vi "Get Channel Data.vi"(5 "Static File Structure":bool, 6 "Tree Location":string, 7 "Relative File Paths":string[](array[string]), 8 "error in (no error)":errorcluster, 9 "Hierarchy":string[](array[string]), 10 "Data Directory":path, 11 "TreeControl in":refnum<vi>) -> (0 "error out":errorcluster, 3 "Tree Selection Data Array":T1[](array[typedef]))   [LabVIEW 2017, in "XTree.xctl"]
doc: "Gets information of all of the channels under a location in the tree."
uses:
  <vilib>/addons/_NIFileIO/XTree/XTree.xctl
  <vilib>/addons/_NIFileIO/XTree/Controls/Tree Selection Data.ctl
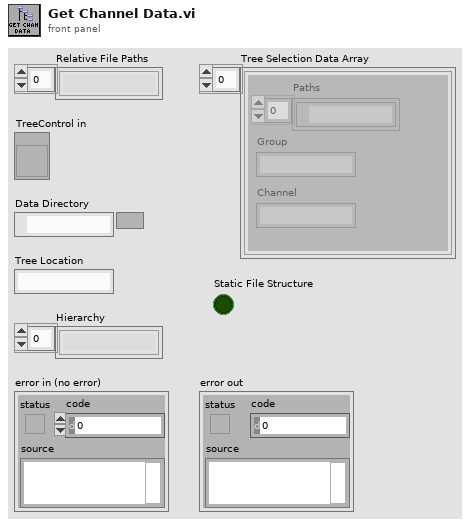
[diagram p1: front panel]
types:
  T1 = typedef "XTree.xctl/Tree Selection Data.ctl" = cluster{"Paths":path[], "Group":string, "Channel":string}
  T2 = enum16{"open", "open or create", "create or replace", "create", "open (read-only)"}
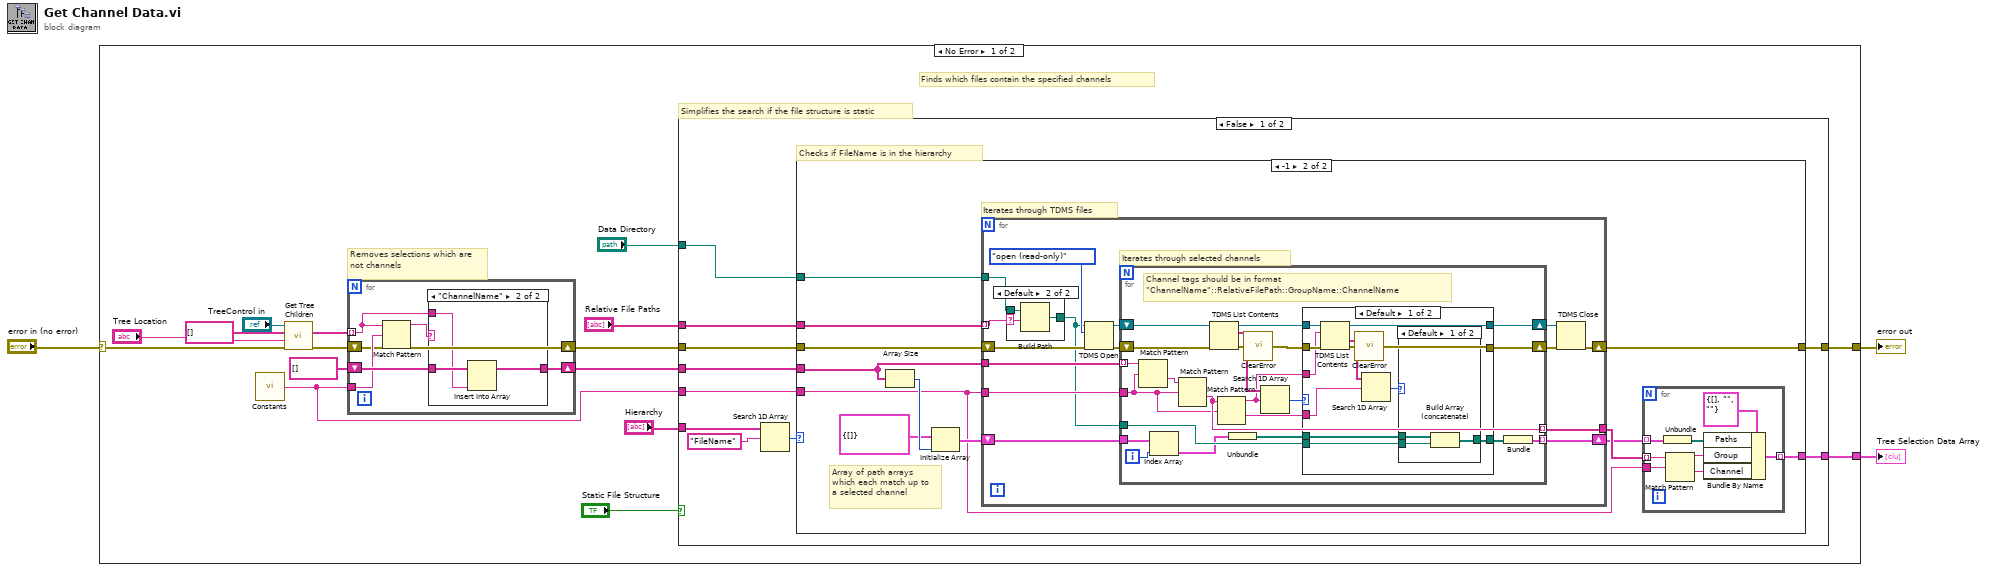
[diagram p0: block diagram]
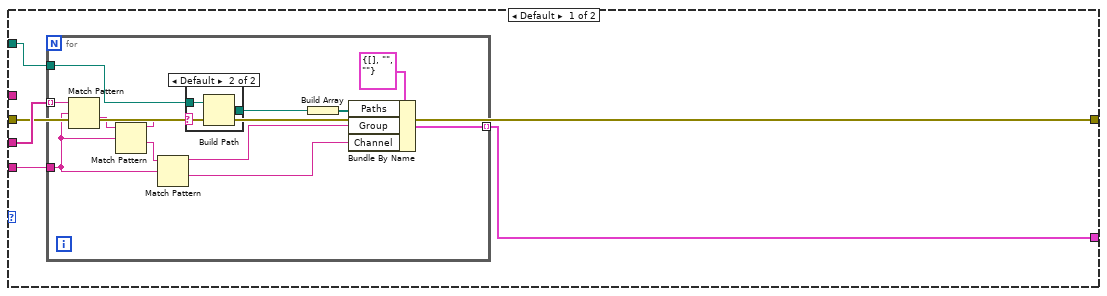
[diagram p2: hidden frame]
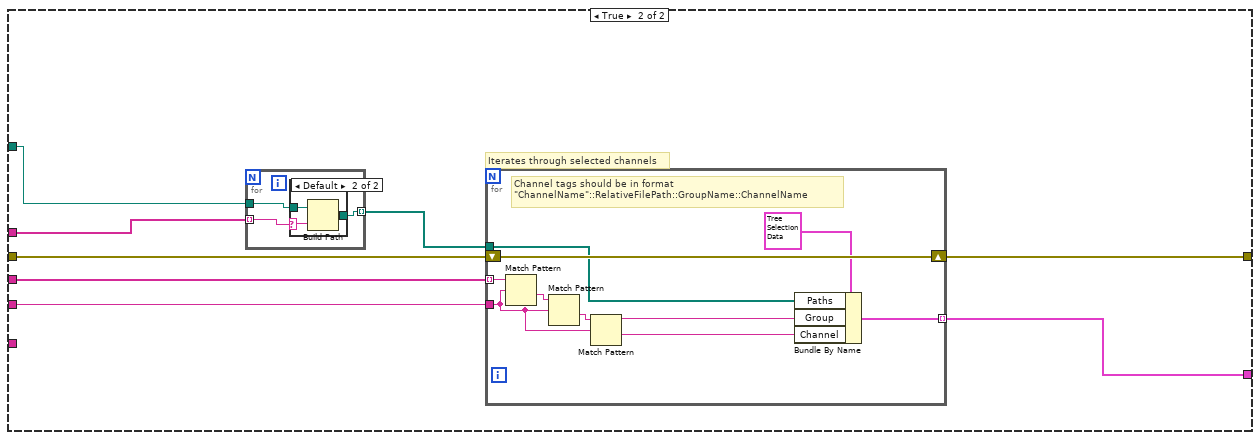
[diagram p7: hidden frame]
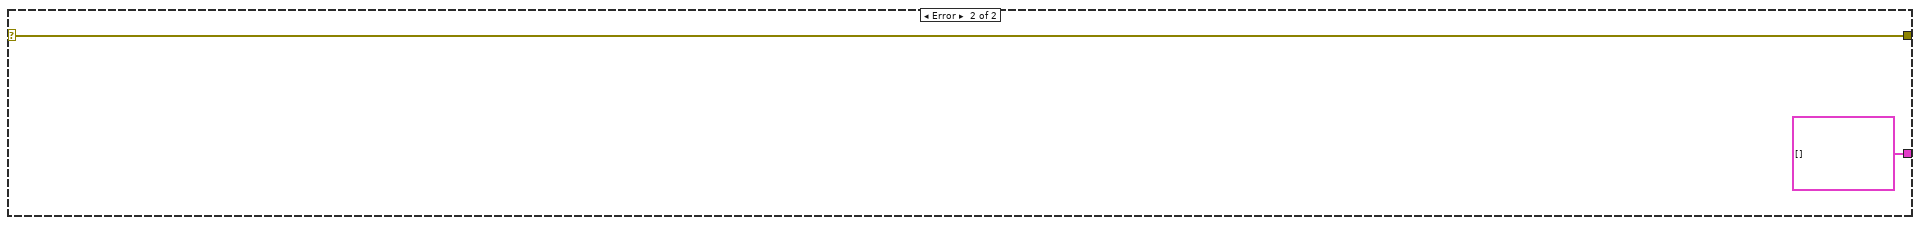
[diagram p10: hidden frame]
diagram:
  n1 = case shown="No Error" "error in (no error)" {
    selector: "error in (no error)" -> [w5 w167]
    tunnel: [w18 w167] -> w3
    tunnel: [w4 T1[] []] -> w1
    frame No Error {
      # "Simplifies the search if the file structure is static"
      # "Finds which files contain the specified channels"
      # "Removes selections which are not channels"
      n2 = call <vilib>:"Constants.vi"() -> ("String Delimeter"=w10:string)  [unwired: 5 in]
      n3 = call <vilib>:"Get Tree Children.vi"("error in (no error)"=w5, "Parent Tag"="Tree Location", "Child Tags In"=string[] [], "File Contents Tree"="TreeControl in") -> ("error out"=w11:errorcluster, "Child Tags Out"=w13:string[])  [unwired: 6 in]
      n4 = for {
        tunnel: w13 -> [w159] mode=indexing
        shift-right: [w160] -> w9
        shift-left: string[] [] -> [w161]
        shift-right: [w156] -> w8
        shift-left: w11 -> [w156]
        tunnel: w10 -> [w158]
        n5 = Match Pattern(string=w159, regular expression=w158) -> (before substring=w157:string)  [unwired: 1 in, 3 out]
        n6 = case shown="\"ChannelName\"" w157 {
          tunnel: w161 -> [w162 w165]
          tunnel: [w162 w164] -> w160
          tunnel: w159 -> [_ w163]
          frame Default {
          }
          frame "ChannelName" {
            n7 = Insert Into Array(array=w165, new element=w163) -> (w164:string[])  [unwired: 1 in]
          }
        }
      }
      n8 = case shown="False" "Static File Structure" {
        tunnel: "Hierarchy" -> [w27 _]
        tunnel: [w26 w132] -> w4
        tunnel: [w25 w138] -> w18
        tunnel: "Data Directory" -> [w24 w137]
        tunnel: "Relative File Paths" -> [w23 w136]
        tunnel: w10 -> [w22 w135]
        tunnel: w9 -> [w21 w134]
        tunnel: w8 -> [w20 w131]
        frame False {
          # "Checks if FileName is in the hierarchy"
          n9 = Search 1D Array(1D array=w27, element="FileName") -> (index of element=w29:i32)  [unwired: 1 in]
          n10 = case shown="-1" w29 {
            tunnel: w23 -> [_ w62]
            tunnel: w20 -> [w30 w61]
            tunnel: w21 -> [w34 w57]
            tunnel: w24 -> [w32 w54]
            tunnel: [w30 w53] -> w25
            tunnel: [w31 w52] -> w26
            tunnel: w22 -> [w33 w51]
            frame Default {
              n11 = for {
                tunnel: w34 -> [w46] mode=indexing
                tunnel: w33 -> [w41]
                tunnel: w32 -> [w37]
                tunnel: [w43] -> w31 mode=indexing
                n12 = Match Pattern(string=w46, regular expression=w41) -> (after substring=w45:string)  [unwired: 1 in, 3 out]
                n13 = Match Pattern(string=w45, regular expression=w41) -> (before substring=w36:string, after substring=w42:string)  [unwired: 1 in, 2 out]
                n14 = Match Pattern(string=w42, regular expression=w41) -> (before substring=w40:string, after substring=w39:string)  [unwired: 1 in, 2 out]
                n15 = case shown="Default" w36 {
                  selector: w36 -> [_ w48]
                  tunnel: w37 -> [w47 w50]
                  tunnel: [w47 w49] -> w35
                  frame "" {
                  }
                  frame Default {
                    n16 = Build Path(base path=w50, name or relative path=w48) -> (appended path=w49:path)
                  }
                }
                n17 = Build Array(w35) -> (w44:path[])
                n18 = Bundle By Name(cluster=T1 {"Paths"=[], "Group"="", "Channel"=""} ("Tree Selection Data"), "Paths"=w44, "Group"=w40, "Channel"=w39) -> (w43:T1)
              }
            }
            frame -1 {
              # "Array of path arrays which each match up to a selected channel"
              # "Iterates through TDMS files"
              n19 = Array Size(array=w57) -> (size(s)=w58:i32)
              n20 = Initialize Array(cluster{path[]} {[]}, w58) -> (w55:cluster{path[]}[])
              n21 = for {
                tunnel: w62 -> [w71] mode=indexing
                shift-right: [w84] -> w53
                shift-left: w61 -> [w74]
                tunnel: w57 -> [w82]
                tunnel: w51 -> [w79]
                shift-right: [w77] -> w59
                shift-left: w55 -> [w78]
                tunnel: [w76] -> w60
                tunnel: w54 -> [w73]
                # "Iterates through selected channels"
                n22 = case shown="Default" w71 {
                  selector: w71 -> [_ w87]
                  tunnel: w73 -> [w86 w89]
                  tunnel: [w86 w88] -> w72
                  frame "" {
                  }
                  frame Default {
                    n23 = Build Path(base path=w89, name or relative path=w87) -> (appended path=w88:path)
                  }
                }
                n24 = TDMS Open(8:w74, 10:T2."open (read-only)" ("operation (0:open)"), 11:w72) -> (0:w75:errorcluster, 3:w80:refnum<k34>)  [unwired: 4 in]
                n25 = for {
                  tunnel: w72 -> [w111]
                  shift-right: [w109] -> w85
                  shift-left: w75 -> [w98]
                  tunnel: w82 -> [w110] mode=indexing
                  tunnel: w79 -> [w100]
                  tunnel: w78 -> [w105]
                  tunnel: [w106] -> w77 mode=indexing
                  tunnel: [w101] -> w76 mode=indexing
                  shift-right: [w91] -> w83
                  shift-left: w80 -> [w99]
                  i -> [w104]
                  # "Channel tags should be in format \n\"ChannelName\"::RelativeFilePath::GroupName::ChannelName"
                  n26 = Match Pattern(string=w110, regular expression=w100) -> (after substring=w102:string)  [unwired: 1 in, 3 out]
                  n27 = Index Array(array=w105, index=w104) -> (element=w103:cluster{path[]})
                  n28 = Match Pattern(string=w102, regular expression=w100) -> (after substring=w101:string)  [unwired: 1 in, 3 out]
                  n29 = TDMS List Contents(4:w98, 7:w99) -> (0:w90:errorcluster, 2:w96:string[], 3:w93:refnum<k34>)  [unwired: 1 in, 1 out]
                  n30 = Match Pattern(string=w101, regular expression=w100) -> (before substring=w94:string, after substring=w95:string)  [unwired: 1 in, 2 out]
                  n31 = Unbundle(w103) -> (w108:path[])
                  n32 = call <vilib>:"ClearError.vi"("error in (no error)"=w90) -> ("error out"=w92:errorcluster)
                  n33 = Search 1D Array(1D array=w96, element=w94) -> (index of element=w97:i32)  [unwired: 1 in]
                  n34 = case shown="Default" w97 {
                    tunnel: [w114 w129] -> w109
                    tunnel: w108 -> [w117 w130]
                    tunnel: w111 -> [w115 _]
                    tunnel: [w116 w130] -> w107
                    tunnel: w95 -> [w118 _]
                    tunnel: w94 -> [w120 _]
                    tunnel: w93 -> [w123 w128]
                    tunnel: w92 -> [w122 w129]
                    tunnel: [w113 w128] -> w91
                    frame Default {
                      n35 = TDMS List Contents(4:w122, 6:w120, 7:w123) -> (0:w112:errorcluster, 1:w119:string[], 3:w113:refnum<k34>)  [unwired: 1 out]
                      n36 = call <vilib>:"ClearError.vi"("error in (no error)"=w112) -> ("error out"=w114:errorcluster)
                      n37 = Search 1D Array(1D array=w119, element=w118) -> (index of element=w121:i32)  [unwired: 1 in]
                      n38 = case shown="Default" w121 {
                        tunnel: w117 -> [w126 w127]
                        tunnel: [w125 w127] -> w116
                        tunnel: w115 -> [w124 _]
                        frame Default {
                          n39 = Build Array (concatenate)(w126, w124) -> (w125:path[])
                        }
                        frame -1 {
                        }
                      }
                    }
                    frame -1 {
                    }
                  }
                  n40 = Bundle(w107) -> (w106:cluster{path[]})  [unwired: 1 in]
                }
                n41 = TDMS Close(8:w85, 11:w83) -> (0:w84:errorcluster)  [unwired: 1 out]
              }
              n42 = for {
                tunnel: w60 -> [w70] mode=indexing
                tunnel: w51 -> [w69]
                tunnel: w59 -> [w68] mode=indexing
                tunnel: [w66] -> w52 mode=indexing
                n43 = Unbundle(w68) -> (w67:path[])
                n44 = Match Pattern(string=w70, regular expression=w69) -> (before substring=w65:string, after substring=w64:string)  [unwired: 1 in, 2 out]
                n45 = Bundle By Name(cluster=T1 {"Paths"=[], "Group"="", "Channel"=""} ("Tree Selection Data"), "Paths"=w67, "Group"=w65, "Channel"=w64) -> (w66:T1)
              }
            }
          }
        }
        frame True {
          # "Iterates through selected channels"
          n46 = for {
            tunnel: w136 -> [w141] mode=indexing
            tunnel: w137 -> [w140]
            tunnel: [w139] -> w133 mode=indexing
            n47 = case shown="Default" w141 {
              selector: w141 -> [_ w143]
              tunnel: w140 -> [w142 w145]
              tunnel: [w142 w144] -> w139
              frame "" {
              }
              frame Default {
                n48 = Build Path(base path=w145, name or relative path=w143) -> (appended path=w144:path)
              }
            }
          }
          n49 = for {
            shift-right: [w151] -> w138
            shift-left: w131 -> [w151]
            tunnel: w134 -> [w155] mode=indexing
            tunnel: w135 -> [w152]
            tunnel: w133 -> [w147]
            tunnel: [w146] -> w132 mode=indexing
            # "Channel tags should be in format \n\"ChannelName\"::RelativeFilePath::GroupName::ChannelName"
            n50 = Match Pattern(string=w155, regular expression=w152) -> (after substring=w154:string)  [unwired: 1 in, 3 out]
            n51 = Match Pattern(string=w154, regular expression=w152) -> (after substring=w153:string)  [unwired: 1 in, 3 out]
            n52 = Match Pattern(string=w153, regular expression=w152) -> (before substring=w149:string, after substring=w148:string)  [unwired: 1 in, 2 out]
            n53 = Bundle By Name(cluster=T1 {"Paths"=[], "Group"="Tachometer", "Channel"="Tach Chan"} ("Tree Selection Data"), "Paths"=w147, "Group"=w149, "Channel"=w148) -> (w146:T1)
          }
        }
      }
    }
    frame Error {
    }
  }
  "error out" <- w3
  "Tree Selection Data Array" <- w1
